vi "LASER_StopAll.vi"(8 "error in":errorcluster, 11 "Constant Output Configuration":T1) -> (0 "error out":errorcluster, 3 "Constant Output Configuration (dup)":T1)   [LabVIEW 2010]
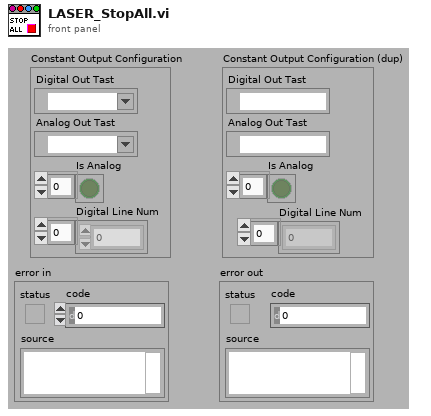
[diagram p1: front panel]
types:
  T1 = cluster{"Digital Out Tast":refnum<k21>, "Analog Out Tast":refnum<k21>, "Is Analog":bool[], "Digital Line Num":u32[]}
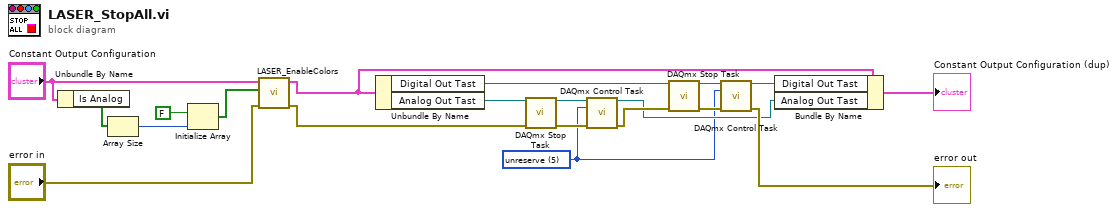
[diagram p0: block diagram]
diagram:
  w12 = 5 items=["verify"=2, "reserve"=4, "commit"=3, "unreserve"=5, "abort"=6] ("action")
  n1 = Unbundle By Name("Constant Output Configuration") -> ("Is Analog"=w3:bool[])
  n2 = Array Size(array=w3) -> (size(s)=w2:i32)
  n3 = Initialize Array(FALSE ("Global Stop"), w2) -> (w1:bool[])
  n4 = call "LASER_EnableColors.vi"("error in"="error in", "Enabled Colors"=w1, "Constant Output Configuration"="Constant Output Configuration") -> ("error out"=w6:errorcluster, "Constant Output Configuration (dup)"=w8:T1)  [unwired: 7 in]
  n5 = Unbundle By Name(w8) -> ("Digital Out Tast"=w10:refnum<k21>, "Analog Out Tast"=w11:refnum<k21>)
  n6 = call <vilib>:"DAQmx Stop Task.vi"("task/channels in"=w11, "error in"=w6) -> ("task out"=w19:refnum<k21>, "error out"=w20:errorcluster)  [unwired: 12 in]
  n7 = call <vilib>:"DAQmx Control Task.vi"("task/channels in"=w19, "action"=w12, "error in"=w20) -> ("task out"=w13:refnum<k21>, "error out"=w16:errorcluster)  [unwired: 11 in]
  n8 = call <vilib>:"DAQmx Stop Task.vi"("task/channels in"=w10, "error in"=w16) -> ("task out"=w18:refnum<k21>, "error out"=w15:errorcluster)  [unwired: 12 in]
  n9 = call <vilib>:"DAQmx Control Task.vi"("task/channels in"=w18, "action"=w12, "error in"=w15) -> ("task out"=w17:refnum<k21>, "error out"=→"error out":errorcluster)  [unwired: 11 in]
  n10 = Bundle By Name(cluster=w8, "Digital Out Tast"=w17, "Analog Out Tast"=w13) -> (→"Constant Output Configuration (dup)":T1)
